vi "Add Attribute - Object.vi"(8 "error in (no error)":errorcluster, 9 "Value":refnum<class "YAML Parser.lvclass">, 10 "Attribute":string, 11 "YAML Parser in":refnum<class "YAML Parser.lvclass">) -> (0 "error out":errorcluster, 3 "YAML Parser out":refnum<class "YAML Parser.lvclass">)   [LabVIEW 2015, in "YAML Parser.lvclass"]
uses:
  YAML Parser.lvclass
  YAML Parser.lvclass/YAML Parser.ctl
panel:
  out "replaced":bool
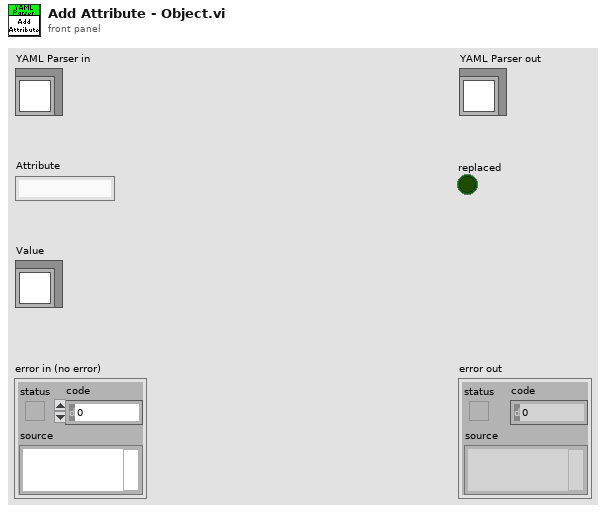
[diagram p1: front panel]
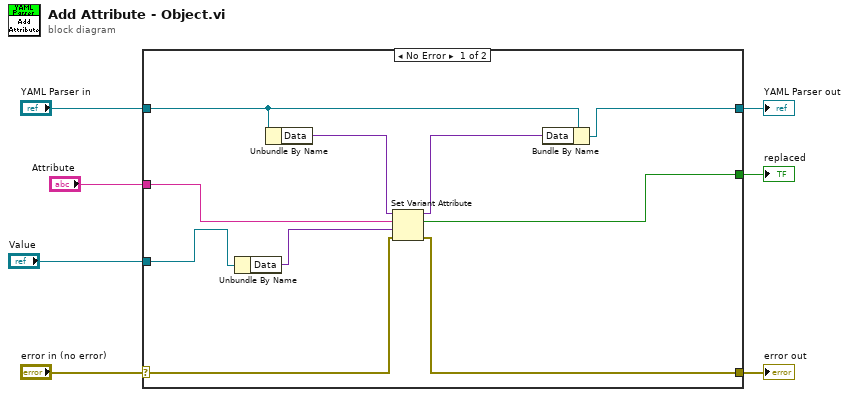
[diagram p0: block diagram]
diagram:
  n1 = case shown="No Error" "error in (no error)" {
    selector: "error in (no error)" -> [w15 w19]
    tunnel: [w14 w19] -> w6
    tunnel: [w17 w18] -> w4
    tunnel: "YAML Parser in" -> [w16 w18]
    tunnel: "Attribute" -> [w11 _]
    tunnel: [w10 _] -> w2
    tunnel: "Value" -> [w9 _]
    frame No Error {
      n2 = Unbundle By Name(w9) -> ("Data"=w8:variant)
      n3 = Unbundle By Name(w16) -> ("Data"=w13:variant)
      n4 = Set Variant Attribute(Variant=w13, name=w11, value=w8, error in=w15) -> (Variant out=w12:variant, replaced=w10:bool, error out=w14:errorcluster)
      n5 = Bundle By Name(cluster=w16, "Data"=w12) -> (w17:refnum<class "YAML Parser.lvclass">)
    }
    frame Error {
    }
  }
  "error out" <- w6
  "YAML Parser out" <- w4
  "replaced" <- w2
